vi "insert_multiple.vi"(7 "connection_reference":T1, 8 "error in (no error)":errorcluster, 10 "value []":dbl[](array[numeric]), 11 "date_time []":dbl[](array[numeric]) format="%<%H:%M:%S%3u %m/%d/%y>T") -> (0 "error out":errorcluster)   [LabVIEW 2015, in "lv-example-postgres.lvlib"]
uses:
  lv-example-postgres.lvlib
  <vilib>/addons/database/Connection.llb/Conn ObjectReference.ctl
  <vilib>/addons/database/Command.llb/Cmd Execute.vi
  <vilib>/addons/database/Recordset.llb/Rec Destroy - Command.vi
  <vilib>/addons/database/Command.llb/Cmd Delete.vi
  <vilib>/addons/database/NI_Database_API.lvlib
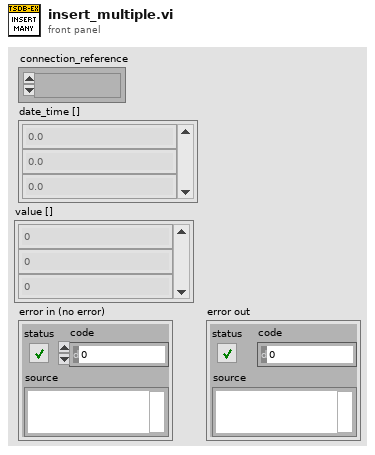
[diagram p1: front panel]
types:
  T1 = typedef "NI_Database_API.lvlib/Conn ObjectReference.ctl" = refnum<k1>
  T2 = typedef "NI_Database_API.lvlib/DB Tools Parameter Info.ctl" = cluster{"parameter name":string, "type":T3, "direction":T4, "value":variant}
  T3 = typedef "NI_Database_API.lvlib/DB Tools DataTypes.ctl" = enum16{"String", "Long (I32)", "Single (SGL)", "Double (DBL)", "Date/Time", "Binary"}
  T4 = typedef "NI_Database_API.lvlib/DB Tools Parameter Dir.ctl" = enum32{"Input", "Output", "Input/Output", "Return Value"}
  T5 = typedef "NI_Database_API.lvlib/Cmd ObjectReference.ctl" = refnum<k1>
  T6 = typedef "NI_Database_API.lvlib/Cmd-Rec Object Reference.ctl" = refnum<k1>
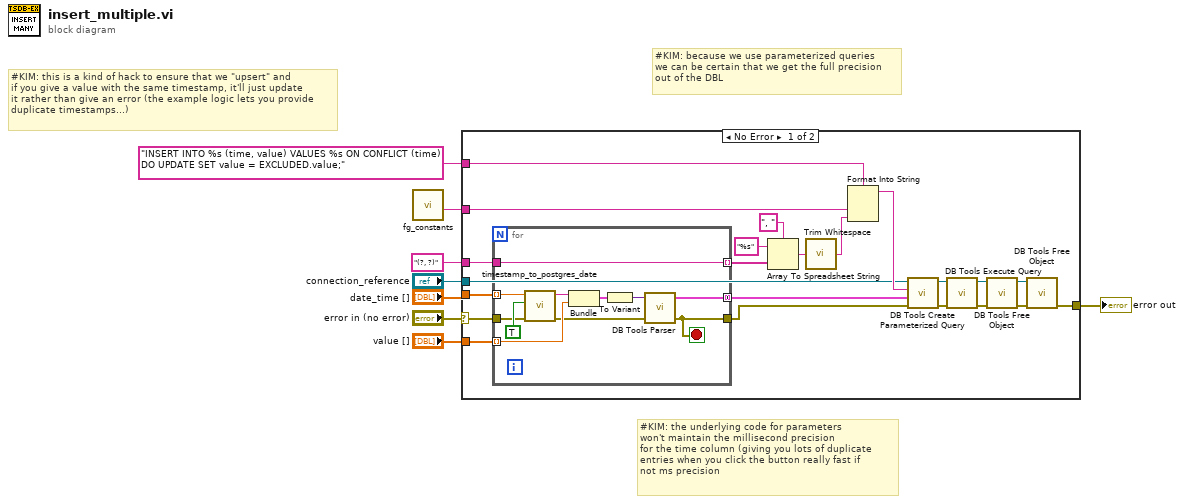
[diagram p0: block diagram]
diagram:
  # "#KIM: this is a kind of hack to ensure that we \"upsert\" and\nif you give a value with the same timestamp, it'll just update\nit rather than give an error (the example logic lets you provide\nduplicate timestamps...)"
  # "#KIM: because we use parameterized queries\nwe can be certain that we get the full precision\nout of the DBL"
  # "#KIM: the underlying code for parameters\nwon't maintain the millisecond precision\nfor the time column (giving you lots of duplicate\nentries when you click the button really fast if\nnot ms precision"
  n1 = call "fg_constants.vi"() -> ("table out"=w2:string)  [unwired: 9 in, 2 out]
  n2 = case shown="No Error" "error in (no error)" {
    selector: "error in (no error)" -> [w12 w42]
    tunnel: "INSERT INTO %s (time, value) VALUES %s ON CONFLICT (time) DO UPDATE SET value = EXCLUDED.value;" ("format string") -> [w30 _]
    tunnel: "value []" -> [w29 _]
    tunnel: "date_time []" -> [w28 _]
    tunnel: w2 -> [w27 _]
    tunnel: "connection_reference" -> [w22 _]
    tunnel: [w21 w42] -> w3
    tunnel: "(?, ?)" ("format string") -> [w9 _]
    frame No Error {
      n3 = for {
        tunnel: w29 -> [w41] mode=indexing
        tunnel: w28 -> [w40] mode=indexing
        tunnel: [w35] -> w11 mode=concatenating
        tunnel: [w31] -> w17 mode=indexing
        tunnel: w12 -> [w37]
        tunnel: [w32] -> w10
        tunnel: w9 -> [w31]
        stop <- w32 stop-if-true
        n4 = call "timestamp_to_postgres_date.vi"("error in (no error)"=w37, "utc"=TRUE, "date_time"=w40) -> ("error out"=w34:errorcluster, "postgres_date"=w39:string)  [unwired: 7 in]
        n5 = Bundle("postgres_date"=w39, "value"=w41) -> (w36:cluster{"postgres_date":string, "value":dbl})  [unwired: 1 in]
        n6 = To Variant(anything=w36) -> (Variant=w33:variant)
        n7 = call <vilib>:"DB Tools Parser.vi"("error in (no error)"=w34, "variant"=w33) -> ("error out"=w32:errorcluster, "parameters"=w35:T2[])  [unwired: 2 in]
      }
      n8 = Array To Spreadsheet String(delimiter (Tab)=", ", array=w17, 3:"%s" ("format string")) -> (spreadsheet string=w14:string)
      n9 = call <vilib>:"Trim Whitespace.vi"("string"=w14) -> ("trimmed string"=w13:string)  [unwired: 1 in]
      n10 = Format Into String(format string=w30, w27, w13) -> (resulting string=w26:string)  [unwired: 2 in, 1 out]
      n11 = call <vilib>:"DB Tools Create Parameterized Query.vi"("error in (no error)"=w10, "parameters"=w11, "SQL query"=w26, "connection reference"=w22) -> ("error out"=w19:errorcluster, "command reference"=w23:T5)  [unwired: 3 in, 1 out]
      n12 = call-poly <vilib>:"DB Tools Execute Query.vi"("error in (no error)"=w19, "command reference"=w23) -> ("error out"=w18:errorcluster, "command-recordset reference"=w24:T6)  [unwired: 6 in]
      n13 = call-poly <vilib>:"DB Tools Free Object.vi"("error in (no error)"=w18, "command-recordset reference"=w24) -> ("error out"=w20:errorcluster, "command reference"=w25:T5)  [unwired: 8 in]
      n14 = call-poly <vilib>:"DB Tools Free Object.vi"("error in (no error)"=w20, "command reference"=w25) -> ("error out"=w21:errorcluster)  [unwired: 8 in, 1 out]
    }
    frame Error {
    }
  }
  "error out" <- w3
